vi "SSC DAQmx Write (Analog 1D Wfm).vi"(0 "DAQmx SSC in":T1[](array[typedef]), 5 "Per Instr Waveforms in":waveform(dbl)[][](array[waveform]), 11 "error in":errorcluster) -> (4 "DAQmx SSC out":T1[](array[typedef]), 15 "error out":errorcluster)   [LabVIEW 2020]
doc: "Writes one or more waveforms to a task that contains one or more analog output channels. The waveform data should be in the same order as SSC."
uses:
  Pin Map/SSC DAQmx.ctl
  <vilib>/DAQmx/write.llb/DAQmx Write (Analog 1D Wfm NChan NSamp).vi
  <vilib>/DAQmx/miscellaneous.llb/DAQmx Fill In Error Info.vi
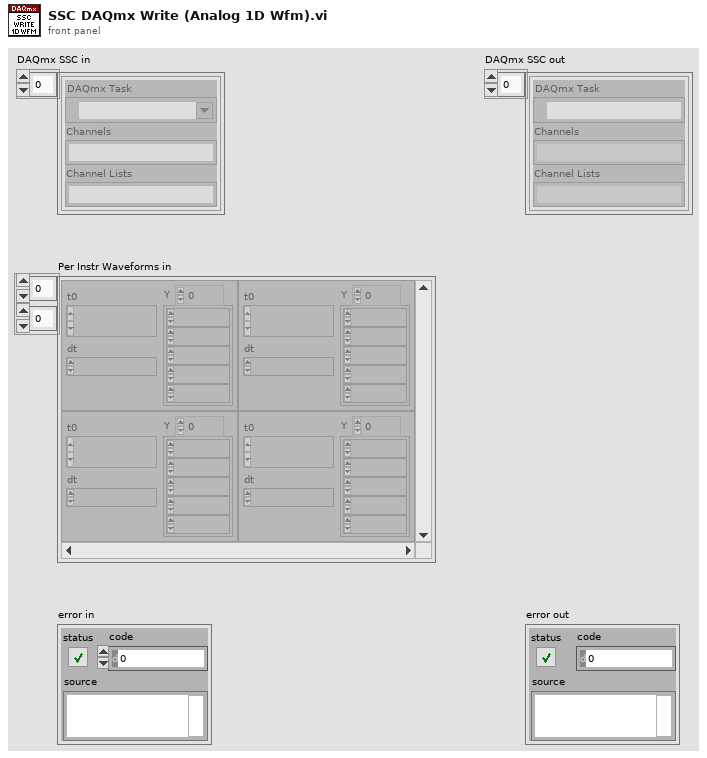
[diagram p1: front panel]
types:
  T1 = typedef "SSC DAQmx.ctl" = cluster{"DAQmx Task ":refnum<k21>, "Channels":string, "Channel Lists":string}
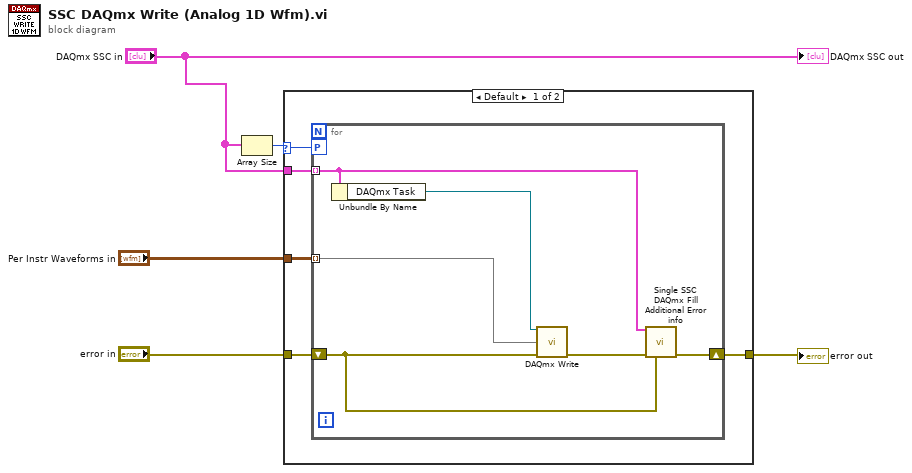
[diagram p0: block diagram]
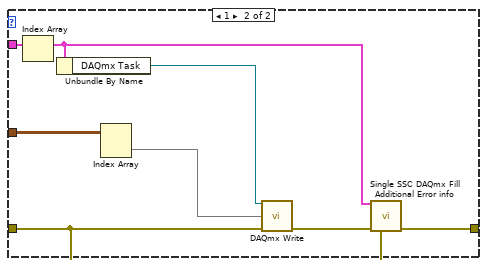
[diagram p2: hidden frame]
diagram:
  n1 = Array Size(array="DAQmx SSC in") -> (size(s)=w3:i32)
  n2 = case shown="Default" w3 {
    selector: w3 -> [w8 _]
    tunnel: [w10 w24] -> w4
    tunnel: "error in" -> [w9 w23]
    tunnel: "DAQmx SSC in" -> [w7 w22]
    tunnel: "Per Instr Waveforms in" -> [w6 w21]
    frame Default {
      n3 = for {
        tunnel: w7 -> [w13] mode=indexing
        workers-P: w8 -> [_]
        shift-right: [w16] -> w10
        shift-left: w9 -> [w15]
        tunnel: w6 -> [w11] mode=indexing
        n4 = Unbundle By Name(w13) -> ("DAQmx Task"=w12:refnum<k21>)
        n5 = call-poly <vilib>:"DAQmx Write.vi"("task/channels in"=w12, "data"=w11, "error in"=w15) -> ("error out"=w14:errorcluster)  [unwired: 10 in, 2 out]
        n6 = call "Single SSC DAQmx Fill Additional Error info.vi"("DAQmx SSC in"=w13, "error in"=w14, "previous error in"=w15) -> ("error out"=w16:errorcluster)  [unwired: 12 in]
      }
    }
    frame 1 {
      n7 = Index Array(array=w22) -> (element=w18:T1)  [unwired: 1 in]
      n8 = Unbundle By Name(w18) -> ("DAQmx Task"=w19:refnum<k21>)
      n9 = Index Array(array=w21) -> (element=w17:waveform(dbl)[])  [unwired: 2 in]
      n10 = call-poly <vilib>:"DAQmx Write.vi"("task/channels in"=w19, "data"=w17, "error in"=w23) -> ("error out"=w20:errorcluster)  [unwired: 10 in, 2 out]
      n11 = call "Single SSC DAQmx Fill Additional Error info.vi"("DAQmx SSC in"=w18, "error in"=w20, "previous error in"=w23) -> ("error out"=w24:errorcluster)  [unwired: 12 in]
    }
  }
  "error out" <- w4
  "DAQmx SSC out" <- "DAQmx SSC in"
